vi "Clear.vi"(8 "error in (no error)":errorcluster, 11 "PSU in":refnum<class "DAQ.lvclass">) -> (0 "error out":errorcluster, 3 "PSU out":refnum<class "DAQ.lvclass">)   [LabVIEW 2020, in "High Level PSU With Tests.lvlib" / "DAQ.lvclass"]
uses:
  DAQ.lvclass
  DAQ.lvclass/DAQ.ctl
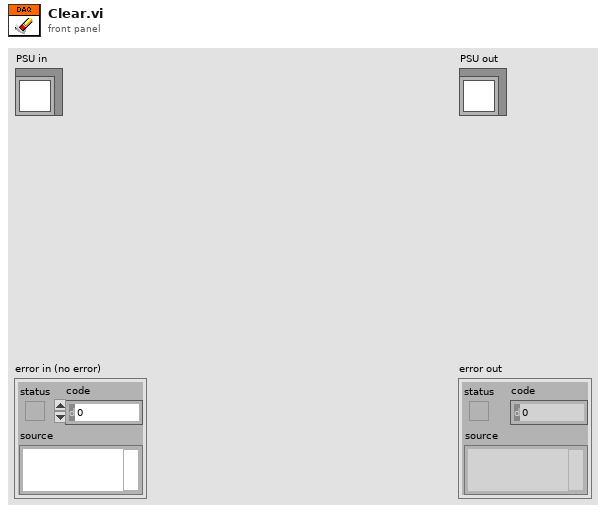
[diagram p1: front panel]
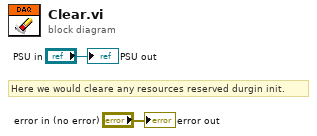
[diagram p0: block diagram]
diagram:
  # "Here we would cleare any resources reserved durgin init."
  "error out" <- "error in (no error)"
  "PSU out" <- "PSU in"
